vi "Initialize_Msg_Queue_FGV.vi"(8 "error in (no error)":errorcluster, 11 "queue in":refnum<queue>) -> (0 "error out":errorcluster)   [LabVIEW 2024, in "Multicom_MP711134-14V.lvlib"]
doc: "ThisVI\n---------------------------------\nInitialize_Queue_FGV\n---------------------------------\n-initialize the FGV Message Queue"
uses:
  Multicom_MP711134-14V.lvlib
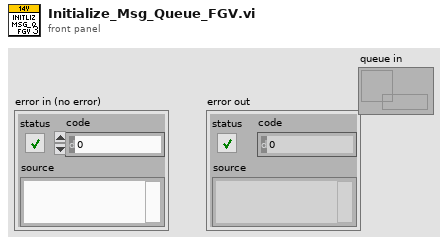
[diagram p1: front panel]
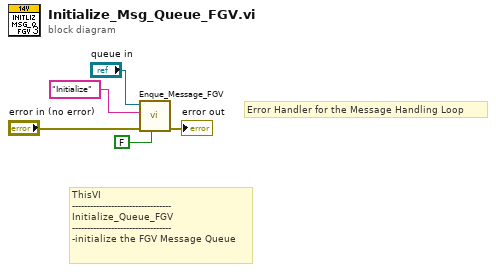
[diagram p0: block diagram]
diagram:
  # "Error Handler for the Message Handling Loop"
  # "ThisVI\n---------------------------------\nInitialize_Queue_FGV\n---------------------------------\n-initialize the FGV Message Queue"
  n1 = call "Enque_Message_FGV.vi"("Priority"=FALSE, "error in (no error)"="error in (no error)", "Message"="Initialize", "queue in"="queue in") -> ("error out"=→"error out":errorcluster)  [unwired: 7 in]
